vi "Eval_BulkMode.vi"(8 "error in (no error)":errorcluster, 11 "muExpr in":refnum<class "mupExpr.lvclass">) -> (0 "error out":errorcluster, 2 "Result":dbl[](array[numeric]) format="%#_13g", 3 "muExpr out":refnum<class "mupExpr.lvclass">)   [LabVIEW 2015, in "mupExpr.lvclass"]
doc: "Evaluates the expression in bulk mode. Returns the array of results.\n\nIf multiple expressions have been input, the result of the last one in the list is returned."
uses:
  mupExpr.lvclass
  mupExpr.lvclass/mupExpr.ctl
  mupLib/mupCheckError.vi
  mupLib/mupLibPath.vi
  <vilib>/Utility/error.llb/Error Cluster From Error Code.vi
  mupLib/mupLib.lvlib
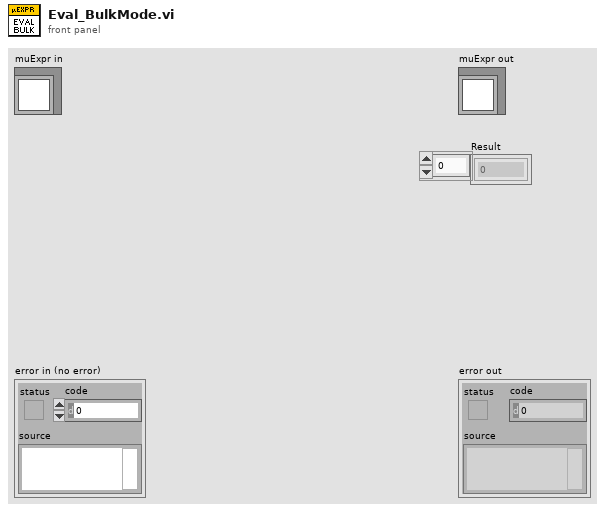
[diagram p1: front panel]
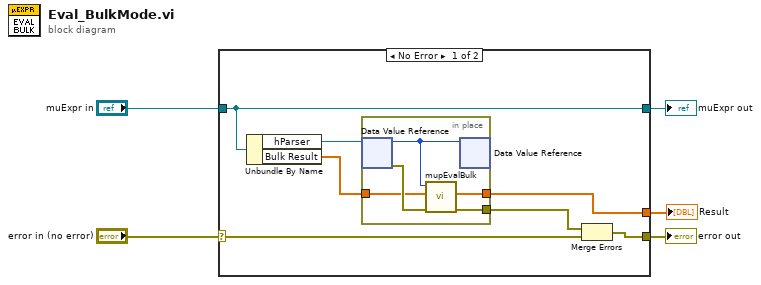
[diagram p0: block diagram]
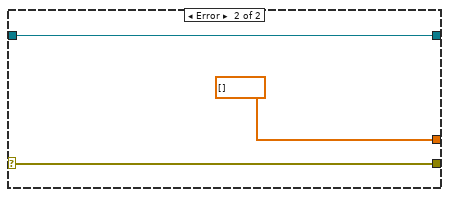
[diagram p2: hidden frame]
diagram:
  n1 = case shown="No Error" "error in (no error)" {
    selector: "error in (no error)" -> [w9 w20]
    tunnel: [w12 w20] -> w4
    tunnel: [w8 w19] -> w2
    tunnel: "muExpr in" -> [w8 w19]
    tunnel: [w7 dbl[] [] ("return type")] -> w1
    frame No Error {
      n2 = Unbundle By Name(w8) -> ("hParser"=w11:refnum<data-value>, "Bulk Result"=w10:dbl[])
      n3 = in-place {
        in-place-border: [w17] -> w6
        in-place-border: [w15] -> w7
        in-place-border: w10 -> [w13]
        n4 = in-place-dvr #1(w11) -> (w14:u64, w16:errorcluster)
        n5 = call "mupEvalBulk.vi"("error in (no error)"=w16, "a_res"=w13, "hParser in"=w14) -> ("error out"=w17:errorcluster, "results"=w15:dbl[])  [unwired: 6 in, 1 out]
        n6 = in-place-dvr #1(w14) -> ()  [unwired: 2 out]
      }
      n7 = Merge Errors(w6, w9) -> (w12:errorcluster)
    }
    frame Error {
    }
  }
  "error out" <- w4
  "muExpr out" <- w2
  "Result" <- w1
